vi "LS330_WriteFile.vi"(8 "error in":errorcluster, 9 "Status IN":cluster{T1, T1}, 10 "current time":timestamp, 11 "File Ref in":refnum<file>) -> (0 "error out":errorcluster, 3 "refnum out":refnum<file>)   [LabVIEW 2021]
uses:
  LS330_Status_Bundle.ctl
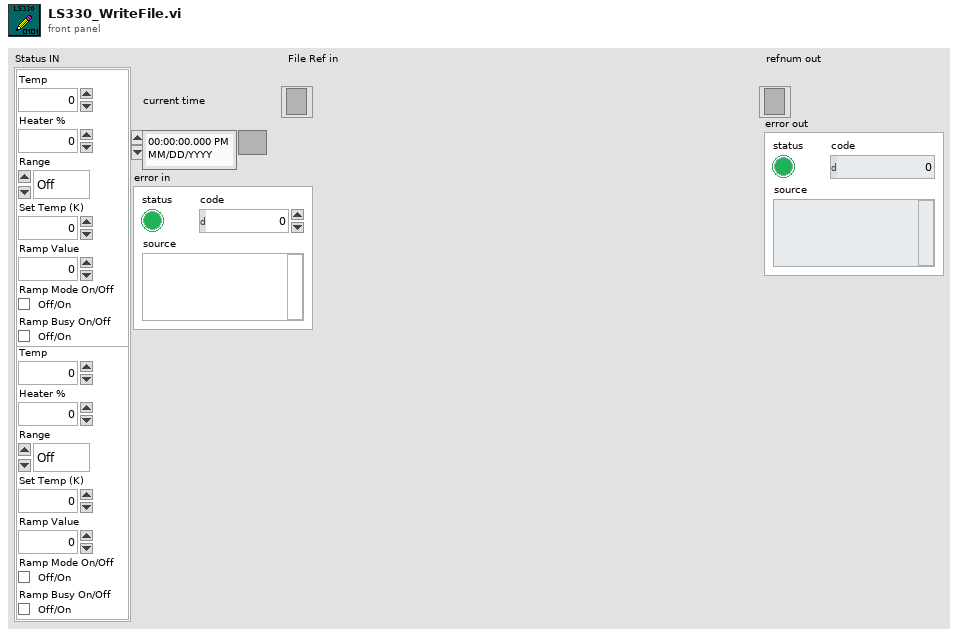
[diagram p1: front panel]
types:
  T1 = typedef "LS330_Status_Bundle.ctl" = cluster{"Temp":dbl, "Heater %":dbl, "Range":enum16{"Off", "Low", "Medium", "High"}, "Set Temp (K)":dbl, "Ramp Value":dbl, "Ramp Mode On/Off":bool, "Ramp Busy On/Off":bool}
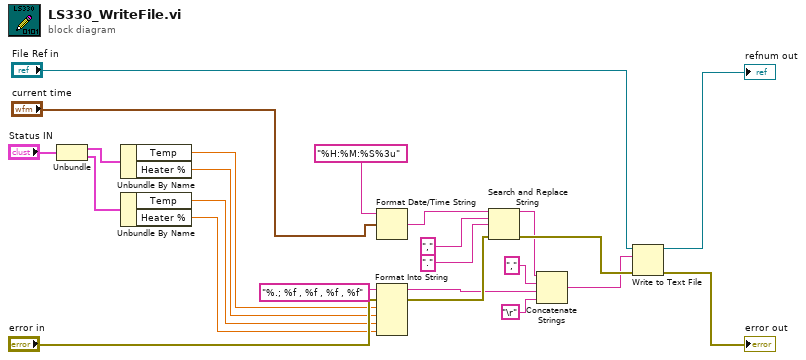
[diagram p0: block diagram]
diagram:
  n1 = Unbundle("Status IN") -> (w23:T1, w22:T1)
  n2 = Unbundle By Name(w23) -> ("Temp"=w19:dbl, "Heater %"=w18:dbl)
  n3 = Unbundle By Name(w22) -> ("Temp"=w17:dbl, "Heater %"=w16:dbl)
  n4 = Format Date/Time String(time format string (%c)="%H:%M:%S%3u", seconds (now)="current time") -> (date/time string=w4:string)  [unwired: 1 in]
  n5 = Format Into String(format string="%.; %f , %f , %f , %f", error in="error in", w19, w18, w17, w16) -> (resulting string=w13:string, error out=w15:errorcluster)  [unwired: 1 in]
  n6 = Search and Replace String(input string=w4, search string=",", replace string="." ("replace string (\"\")"), error in=w15) -> (result string=w5:string, error out=w11:errorcluster)  [unwired: 4 in, 2 out]
  n7 = Concatenate Strings(w5, ",", w13, "\r") -> (w10:string)
  n8 = Write to Text File(file (use dialog)="File Ref in", text=w10, error in=w11) -> (refnum out=→"refnum out":refnum<file>, error out=→"error out":errorcluster)  [unwired: 1 in, 1 out]
